vi "BB_CameraSet Brightness.vi"(8 "error in (no error)":errorcluster, 10 "Brightness":i32=50 min=0 max=100, 11 "Camera Address":string) -> (0 "error out":errorcluster, 3 "Camera Address Out":string)   [LabVIEW 2015]
doc: "Specifies the brightness setting of the camera you specify.\n\nThis software is licensed. Open the labview\\readme\\WPI Robotics Library Open Source License.txt file for more information."
uses:
  <vilib>/Rock Robotics/WPI/Camera/WPI_CameraSettings Operations.ctl
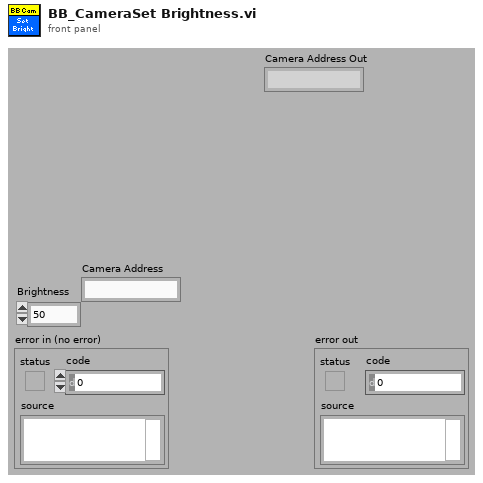
[diagram p1: front panel]
types:
  T1 = typedef "WPI_CameraSettings Operations.ctl" = enum16{"Udate FPS", "Update Compression", "Update Size", "Update White Balance", "Update Brightness", "Update Sharpness", "Update Exposure", "Update Exposure Value", "Update Color Level", "Update Exp Priority", "Update Color Enable", "Update JPG", "Update MJPG", "Read and Clear", "Read", "Init"}
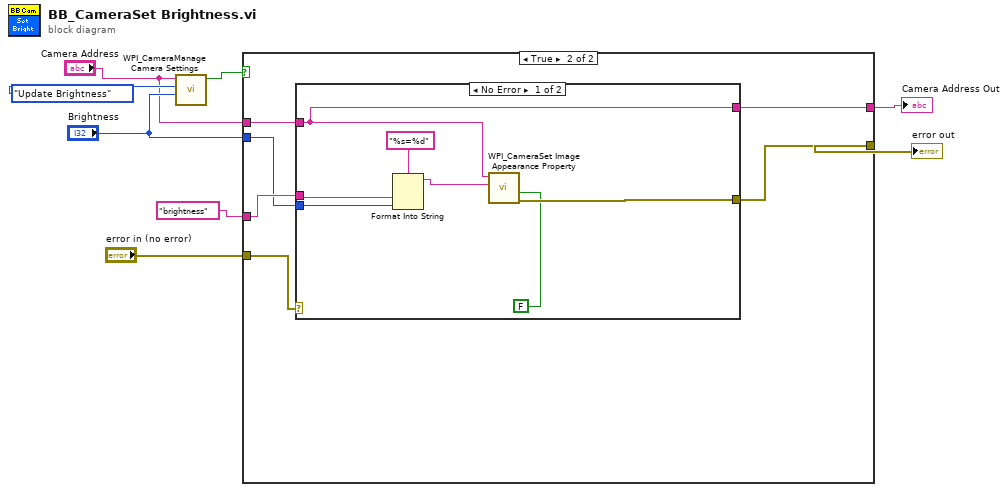
[diagram p0: block diagram]
diagram:
  n1 = call <vilib>:"WPI_CameraManage Camera Settings.vi"("Value"="Brightness", "Operation"=WPI_CameraSettings_Operations."Update Brightness", "Camera IP"="Camera Address") -> ("Changed"=w4:bool)  [unwired: 7 in, 1 out]
  n2 = case shown="True" w4 {
    tunnel: "brightness" ("Property Name") -> [_ w14]
    tunnel: "error in (no error)" -> [w10 w15]
    tunnel: [w10 w16] -> w6
    tunnel: "Brightness" -> [_ w13]
    tunnel: "Camera Address" -> [w9 w12]
    tunnel: [w9 w11] -> w1
    frame False {
    }
    frame True {
      n3 = case shown="No Error" w15 {
        selector: w15 -> [_ w25]
        tunnel: [w20 w25] -> w16
        tunnel: w14 -> [w23 _]
        tunnel: w13 -> [w22 _]
        tunnel: w12 -> [w17 w24]
        tunnel: [w17 w24] -> w11
        frame No Error {
          n4 = Format Into String(format string="%s=%d", w23, w22) -> (resulting string=w19:string)  [unwired: 2 in, 1 out]
          n5 = call <vilib>:"WPI_CameraSet Image Appearance Property.vi"("Appearance"=FALSE, "Prop String"=w19, "address"=w17) -> ("error out"=w20:errorcluster)  [unwired: 8 in]
        }
        frame Error {
        }
      }
    }
  }
  "error out" <- w6
  "Camera Address Out" <- w1
